vi "MainRIOJuan.vi"() -> ()   [LabVIEW 2020]
uses:
  Type Definitions/Acelerometer data--cluster.ctl
  Type Definitions/Shared.lvlib
  <vilib>/PantherLAB/Firebase API/PantherLAB_lib_Filtering Parameters--cluster.ctl
  <vilib>/PantherLAB/Firebase API/PantherLAB_lib_firebase.lvclass
  a087fea8-a487-4c1c-8a8b-15f205e78756.vi
  <vilib>/JDP Science/JSONtext/JSONtext.lvlib
  c90b4970-0cb1-4ed8-a3e8-abf7f56642d0.vi
  079ee137-338a-4224-8d27-3950f07d8dd5.vi
  Type Definitions/RIOData--cluster.ctl
panel:
  in  "Get All":bool
  in  "Get5":bool
  out "JSON String":string
  in  "Get Newest":bool
  in  "Delete":bool
  in  "Password":string
  in  "Email":string
  in  "Log In":bool
  in  "Sign In":bool
  out "Newest":T1
  out "Data out":T1[](array[typedef])
  out "My RIO Acelerometer":T2(graph)
  # "To add an authenticated user\nto your Real Time Database"
  # "If you are already authenticated\nand you want to start using\nyour Database"
  # "Warning:\nThis button will delete all the data\nunder Post EndPoint"
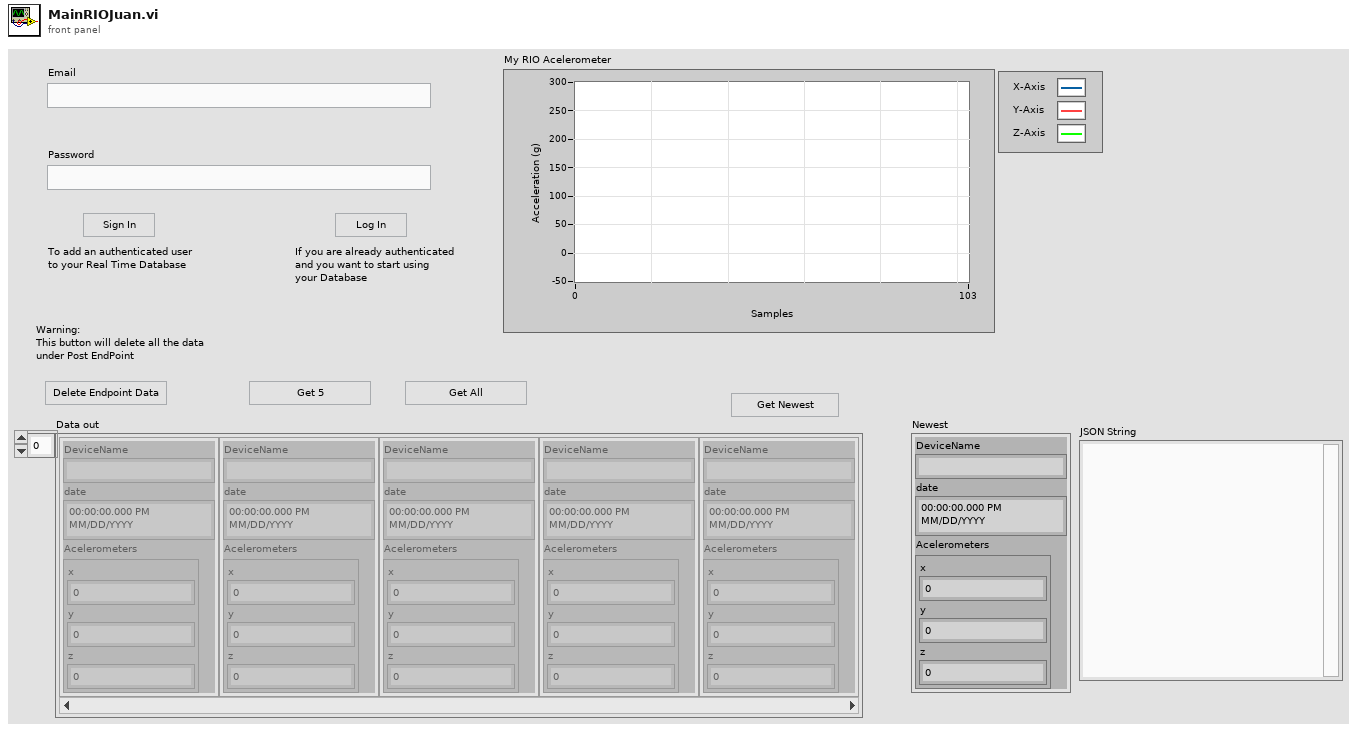
[diagram p1: front panel]
types:
  T1 = typedef "Shared.lvlib/RIOData--cluster.ctl" = cluster{"DeviceName":string, "date":timestamp, "Acelerometers":cluster{"x":dbl, "y":dbl, "z":dbl}}
  T2 = typedef "Shared.lvlib/Acelerometer data--cluster.ctl" = cluster{"X-Axis":dbl, "Y-Axis":dbl, "Z-Axis":dbl}
  T3 = cluster{"Read Access":enum8{"Allowed", "Required", "None"}, "Write Access":enum8{"Allowed", "Required", "None"}}
  T4 = typedef "PantherLAB_lib_firebase.lvclass/PantherLAB_lib_Filtering Parameters--cluster.ctl" = cluster{"Filtering Param":string, "Argument":string}
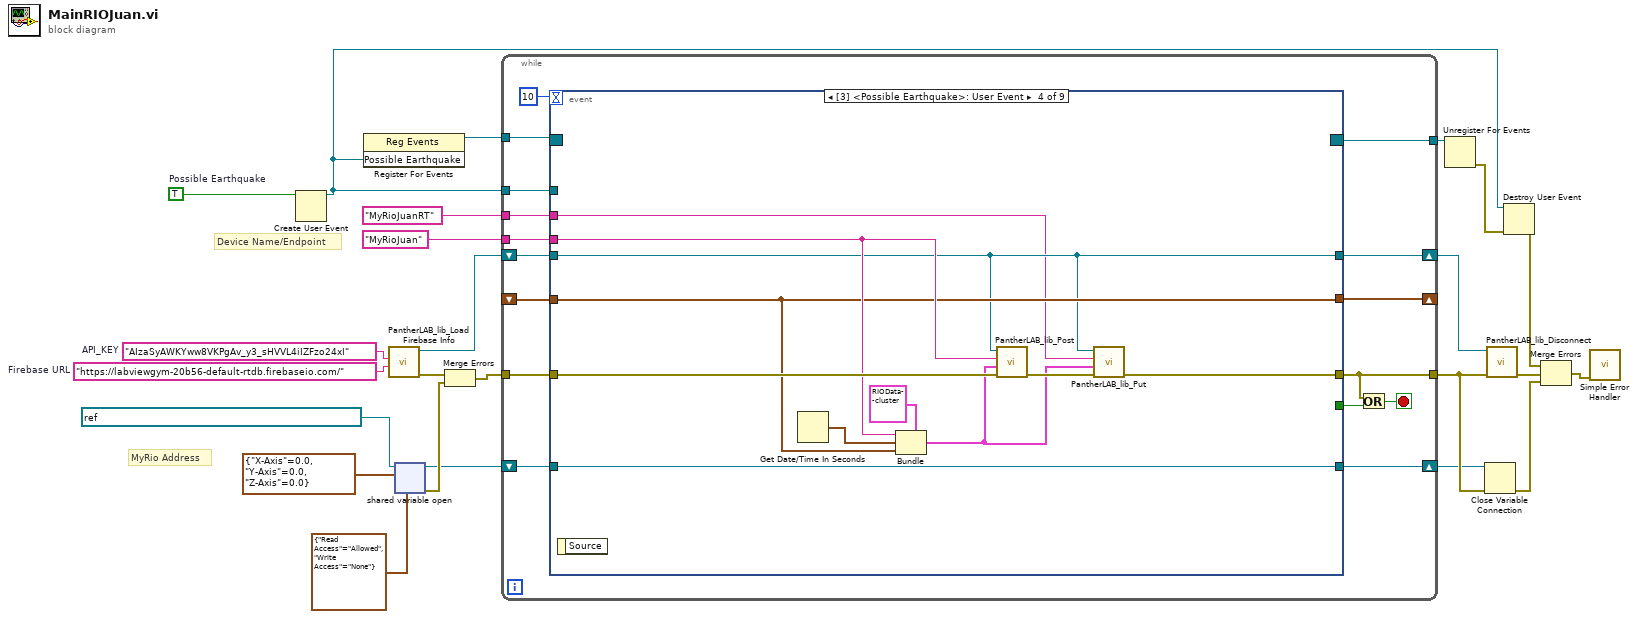
[diagram p0: block diagram]
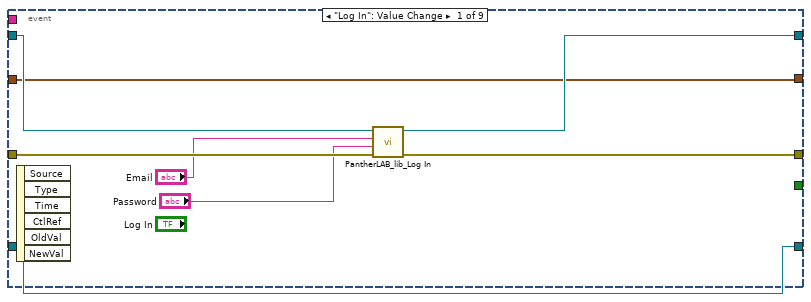
[diagram p2: hidden frame]
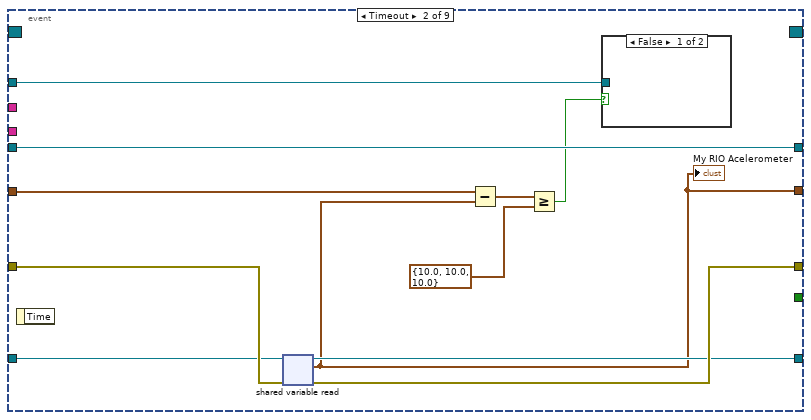
[diagram p3: hidden frame]
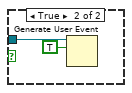
[diagram p4: hidden frame]
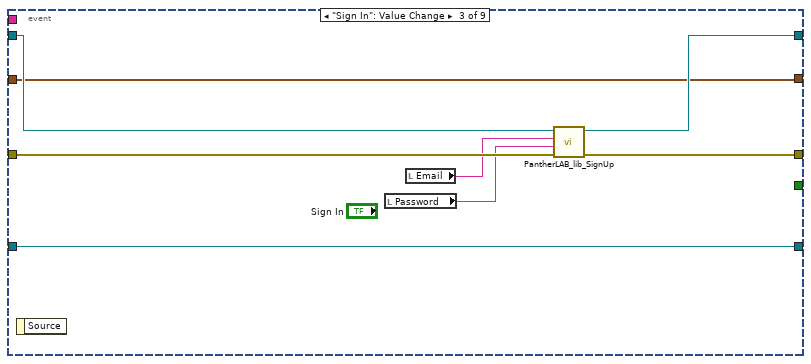
[diagram p5: hidden frame]
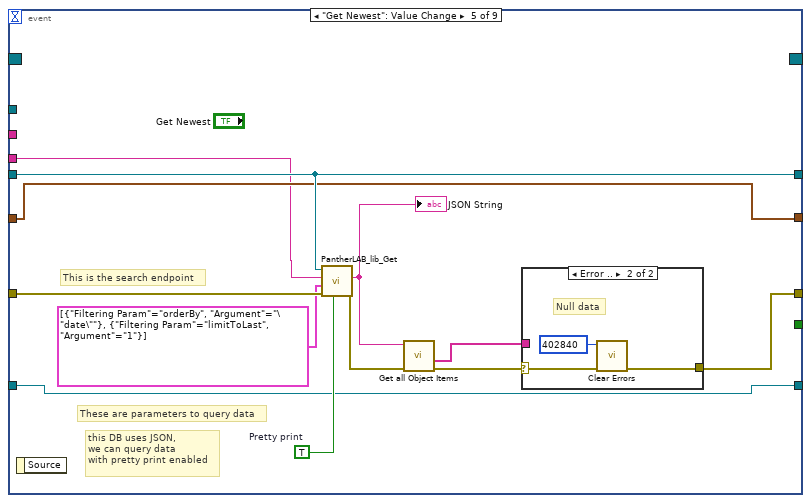
[diagram p6: hidden frame]
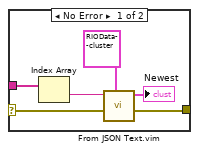
[diagram p7: hidden frame]
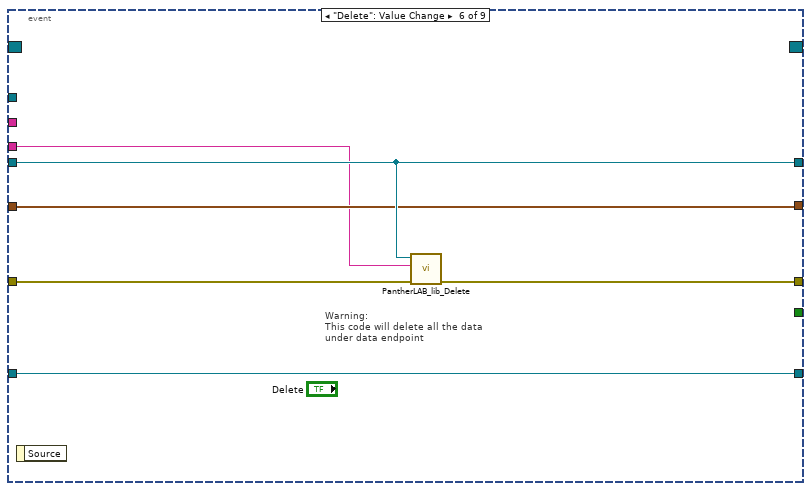
[diagram p8: hidden frame]
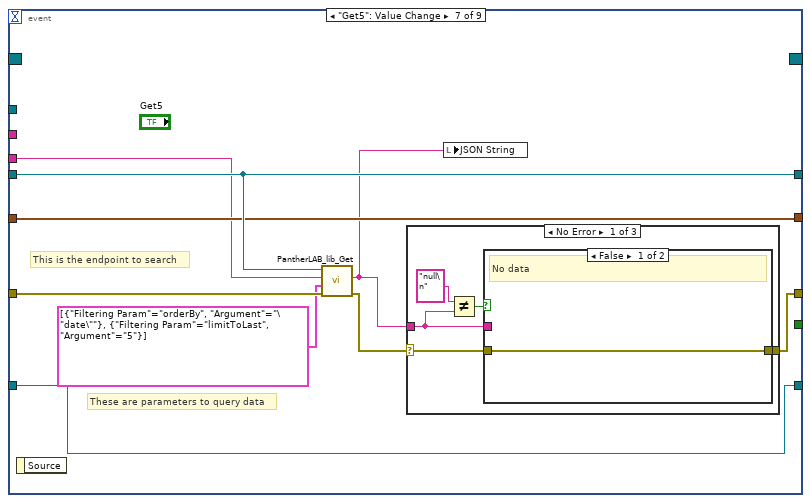
[diagram p9: hidden frame]
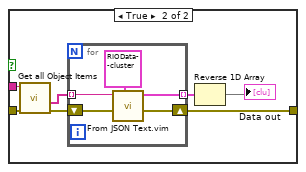
[diagram p10: hidden frame]
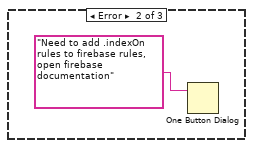
[diagram p11: hidden frame]
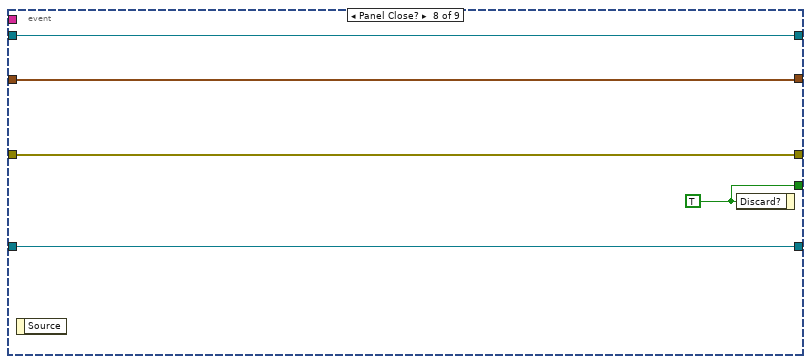
[diagram p13: hidden frame]
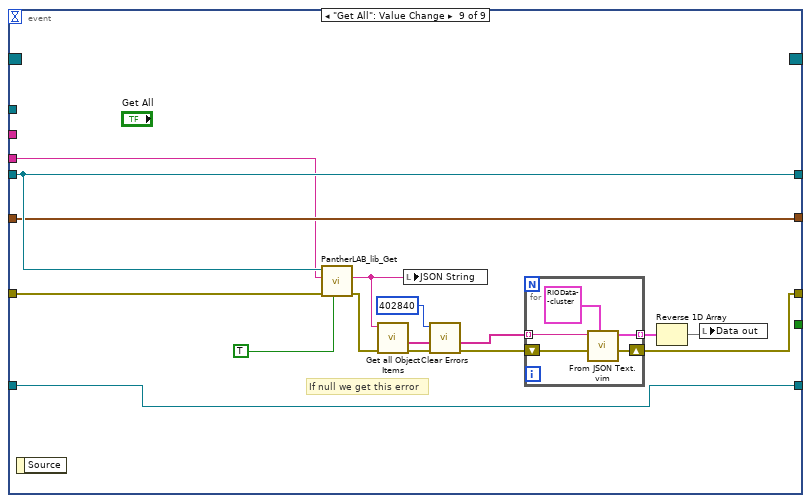
[diagram p14: hidden frame]
diagram:
  w5 = TRUE  # Possible Earthquake
  w10 = "AIzaSyAWKYww8VKPgAv_y3_sHVVL4iIZFzo24xI"  # API_KEY
  w9 = "https://labviewgym-20b56-default-rtdb.firebaseio.com/"  # Firebase URL
  # "MyRio Address"
  # "Device Name/Endpoint"
  n1 = Create User Event(user event datatype=w5) -> (user event=w3:refnum<user-event>)  [unwired: 1 in, 1 out]
  n2 = register-events(w3) -> (reference out=w6:refnum<event-registration>)  [unwired: 2 in, 1 out]
  n3 = call <vilib>:"PantherLAB_lib_Load Firebase Info.vi"("Firebase URL"=w9, "API_KEY"=w10) -> ("error out"=w23:errorcluster, "firebase out"=w11:refnum<class "PantherLAB_lib_firebase.lvclass">)  [unwired: 8 in]
  n4 = shared-variable-open(refnum<k21> "ni.var.psp://mjolnir/MyRIO Data/Accelerometer" ("shared variable refnum in"), T2 {"X-Axis"=0.0, "Y-Axis"=0.0, "Z-Axis"=0.0} ("Acceleration"), T3 {"Read Access"=enum."Allowed", "Write Access"=enum."None"} ("access")) -> (w8:refnum<k21>, w21:errorcluster)  [unwired: 1 in]
  n5 = Merge Errors(w23, w21) -> (w22:errorcluster)
  n6 = while {
    tunnel: w22 -> [w40]
    tunnel: [w39] -> w20
    shift-right: [w35] -> w12
    shift-left: w11 -> [w36]
    shift-right: [w32] -> w7
    shift-left: w8 -> [w33]
    tunnel: w6 -> [w31]
    tunnel: w3 -> [w30]
    shift-right: [w29] -> _
    shift-left: _ -> [w28]
    tunnel: [w27] -> w4
    tunnel: "MyRioJuan" -> [w26]
    tunnel: "MyRioJuanRT" -> [w25]
    stop <- w37 stop-if-true
    n7 = event shown="[3] <Possible Earthquake>: User Event" {
      selector: w31 -> [_ _ _ _ _ _ _ _ _]
      dyn-events: [_ _ _ _ _ _ _ _ _] -> w27
      timeout: 10 -> [_ _ _ _ _ _ _ _ _]
      tunnel: w40 -> [w48 w59 w69 w80 w92 w107 w116 w141 w156]
      tunnel: [w47 w58 w68 w73 w90 w106 w114 w141 w153] -> w39
      tunnel: [_ _ _ _ _ _ _ w139 _] -> w38
      tunnel: w36 -> [w44 w57 w65 w72 w86 w105 w112 w140 w146]
      tunnel: [w43 w57 w64 w72 w86 w105 w112 w140 w146] -> w35
      tunnel: w33 -> [w42 w56 w63 w78 w85 w104 w111 w138 w145]
      tunnel: [w42 w55 w63 w78 w85 w104 w111 w138 w145] -> w32
      tunnel: w30 -> [_ w52 _ _ _ _ _ _ _]
      tunnel: [w41 w50 w62 w74 w84 w103 w110 w137 w144] -> w29
      tunnel: w28 -> [w41 w51 w62 w74 w84 w103 w110 w137 w144]
      tunnel: w26 -> [_ _ _ w77 w83 w102 w109 _ w143]
      tunnel: w25 -> [_ _ _ w71 _ _ _ _ _]
      event "Log In": Value Change {
        n8 = event-data() -> ()  [unwired: 1 in, 6 out]
        n9 = call-dynamic "PantherLAB_lib_Log In.vi"("error in"=w48, "password"="Password", "email"="Email", "firebase in"=w44) -> ("error out"=w47:errorcluster, "firebase out"=w43:refnum<class "PantherLAB_lib_firebase.lvclass">)  [unwired: 6 in]
      }
      event Timeout {
        n10 = event-data() -> ()  [unwired: 1 in, 1 out]
        n11 = shared-variable-read(w56, w59) -> (w55:refnum<k21>, w58:errorcluster, w50:T2)  [unwired: 1 out]
        "My RIO Acelerometer" <- w50
        n12 = Subtract(x=w51, y=w50) -> (x-y=w54:T2)
        n13 = Greater Or Equal?(x=w54, y=T2 {"X-Axis"=10.0, "Y-Axis"=10.0, "Z-Axis"=10.0} ("x")) -> (x >= y?=w49:bool)
        n14 = case shown="False" w49 {
          tunnel: w52 -> [_ w61]
          frame False {
          }
          frame True {
            n15 = Generate User Event(user event=w61, event data cluster=TRUE ("event data")) -> ()  [unwired: 2 in, 2 out]
          }
        }
      }
      event "Sign In": Value Change {
        n16 = event-data() -> ()  [unwired: 1 in, 1 out]
        n17 = local read "Password"() -> (w67:string)
        n18 = local read "Email"() -> (w66:string)
        n19 = call-dynamic "PantherLAB_lib_SignUp.vi"("error in"=w69, "password"=w67, "email"=w66, "firebase in"=w65) -> ("error out"=w68:errorcluster, "firebase out"=w64:refnum<class "PantherLAB_lib_firebase.lvclass">)  [unwired: 6 in]
      }
      event User Event {
        n20 = event-data() -> ()  [unwired: 1 in, 1 out]
        n21 = Get Date/Time In Seconds() -> (seconds since 1Jan1904=w76:timestamp)
        n22 = Bundle(cluster=T1 {"DeviceName"="", "date"=timestamp(0 s since 1904-01-01), "Acelerometers"={"x"=0.0, "y"=0.0, "z"=0.0}} ("output cluster"), "DeviceName"=w77, "date"=w76, "Acelerometers"=w74) -> (w70:T1)
        n23 = call-dynamic "PantherLAB_lib_Post.vi"("error in"=w80, "Anything"=w70, "endPoint"=w77, "firebase in"=w72) -> ("error out"=w79:errorcluster)  [unwired: 6 in, 1 out]
        n24 = call-dynamic "PantherLAB_lib_Put.vi"("error in"=w79, "Anything"=w70, "endPoint"=w71, "firebase in"=w72) -> ("error out"=w73:errorcluster)  [unwired: 6 in, 1 out]
      }
      event "Get Newest": Value Change {
        w87 = TRUE  # Pretty print
        # "this DB uses JSON,\nwe can query data\nwith pretty print enabled"
        # "These are parameters to query data"
        # "This is the search endpoint"
        n25 = event-data() -> ()  [unwired: 1 in, 1 out]
        n26 = call-dynamic "PantherLAB_lib_Get.vi"("Pretty print"=w87, "error in"=w92, "Filtering Params"=T4[] [{"Filtering Param"="orderBy", "Argument"="\"date\""}, {"Filtering Param"="limitToLast", "Argument"="1"}], "endPoint"=w83, "firebase in"=w86) -> ("error out"=w91:errorcluster, "Json String"=w88:string)  [unwired: 5 in]
        "JSON String" <- w88
        n27 = call <vilib>:"Get all Object Items.vi"("error in (no error)"=w91, "JSON"=w88) -> ("error out"=w82:errorcluster, "<JSON>"=w81:string[])  [unwired: 6 in, 2 out]
        n28 = case shown="Error .." w82 {
          selector: w82 -> [w98 w101]
          tunnel: [w97 w100] -> w90
          tunnel: w81 -> [w96 _]
          frame No Error {
            n29 = Index Array(array=w96) -> (element=w95:string)  [unwired: 1 in]
            n30 = call "From JSON Text.vim"("Data Type and Default Value"=T1 {"DeviceName"="", "date"=timestamp(0 s since 1904-01-01), "Acelerometers"={"x"=0.0, "y"=0.0, "z"=0.0}} ("Array"), "error in (no error)"=w98, "JSON"=w95) -> ("error out"=w97:errorcluster, "Data out"=→"Newest":T1)  [unwired: 7 in]
          }
          frame Error {
            # "Null data"
            n31 = call <vilib>:"Clear Errors.vi"("error in (no error)"=w101, "specific error code to clear (0: all)"=402840) -> ("error out"=w100:errorcluster)  [unwired: 4 in, 1 out]
          }
        }
      }
      event "Delete": Value Change {
        # "Warning:\nThis code will delete all the data\nunder data endpoint"
        n32 = event-data() -> ()  [unwired: 1 in, 1 out]
        n33 = call-dynamic "PantherLAB_lib_Delete.vi"("error in"=w107, "endPoint"=w102, "firebase in"=w105) -> ("error out"=w106:errorcluster)  [unwired: 7 in, 1 out]
      }
      event "Get5": Value Change {
        # "This is the endpoint to search"
        # "These are parameters to query data"
        n34 = event-data() -> ()  [unwired: 1 in, 1 out]
        n35 = call-dynamic "PantherLAB_lib_Get.vi"("error in"=w116, "Filtering Params"=T4[] [{"Filtering Param"="orderBy", "Argument"="\"date\""}, {"Filtering Param"="limitToLast", "Argument"="5"}], "endPoint"=w109, "firebase in"=w112) -> ("error out"=w115:errorcluster, "Json String"=w108:string)  [unwired: 6 in]
        n36 = case shown="No Error" w115 {
          selector: w115 -> [w121 _ w136]
          tunnel: [w120 _ w136] -> w114
          tunnel: w108 -> [w117 _ _]
          frame No Error {
            n37 = Not Equal?(x="null\n" ("Display"), y=w117) -> (x != y?=w118:bool)
            n38 = case shown="False" w118 {
              tunnel: w121 -> [w122 w128]
              tunnel: [w122 w127] -> w120
              tunnel: w117 -> [_ w124]
              frame False {
                # "No data"
              }
              frame True {
                n39 = call <vilib>:"Get all Object Items.vi"("error in (no error)"=w128, "JSON"=w124) -> ("error out"=w129:errorcluster, "<JSON>"=w126:string[])  [unwired: 6 in, 2 out]
                n40 = for {
                  tunnel: w126 -> [w132] mode=indexing
                  shift-right: [w133] -> w127
                  shift-left: w129 -> [w134]
                  tunnel: [w131] -> w125 mode=indexing
                  n41 = call "From JSON Text.vim"("Data Type and Default Value"=T1 {"DeviceName"="", "date"=timestamp(0 s since 1904-01-01), "Acelerometers"={"x"=0.0, "y"=0.0, "z"=0.0}} ("RioData"), "error in (no error)"=w134, "JSON"=w132) -> ("error out"=w133:errorcluster, "Data out"=w131:T1)  [unwired: 7 in]
                }
                n42 = Reverse 1D Array(array=w125) -> (reversed array=→"Data out":T1[])
              }
            }
          }
          frame Error {
            n43 = One Button Dialog(message="Need to add .indexOn rules to firebase rules, open firebase documentation") -> ()  [unwired: 1 in, 1 out]
          }
          frame Default {
          }
        }
        n44 = local write "JSON String"(w108) -> ()
      }
      event Panel Close? {
        w139 = TRUE ("Discard?")
        n45 = event-data() -> ()  [unwired: 1 in, 1 out]
        n46 = event-data("Discard?"=w139) -> ()  [unwired: 1 in, 1 out]
      }
      event "Get All": Value Change {
        # "If null we get this error"
        n47 = event-data() -> ()  [unwired: 1 in, 1 out]
        n48 = call-dynamic "PantherLAB_lib_Get.vi"("Pretty print"=TRUE, "error in"=w156, "endPoint"=w143, "firebase in"=w146) -> ("error out"=w154:errorcluster, "Json String"=w149:string)  [unwired: 6 in]
        n49 = call <vilib>:"Get all Object Items.vi"("error in (no error)"=w154, "JSON"=w149) -> ("error out"=w155:errorcluster, "<JSON>"=w151:string[])  [unwired: 6 in, 2 out]
        n50 = local write "JSON String"(w149) -> ()
        n51 = call <vilib>:"Clear Errors.vi"("error in (no error)"=w155, "specific error code to clear (0: all)"=402840) -> ("error out"=w152:errorcluster)  [unwired: 4 in, 1 out]
        n52 = for {
          tunnel: w151 -> [w159] mode=indexing
          shift-right: [w160] -> w153
          shift-left: w152 -> [w161]
          tunnel: [w158] -> w150 mode=indexing
          n53 = call "From JSON Text.vim"("Data Type and Default Value"=T1 {"DeviceName"="", "date"=timestamp(0 s since 1904-01-01), "Acelerometers"={"x"=0.0, "y"=0.0, "z"=0.0}} ("RioData"), "error in (no error)"=w161, "JSON"=w159) -> ("error out"=w160:errorcluster, "Data out"=w158:T1)  [unwired: 7 in]
        }
        n54 = Reverse 1D Array(array=w150) -> (reversed array=w142:T1[])
        n55 = local write "Data out"(w142) -> ()
      }
    }
    n56 = Or(x=w39, y=w38) -> (x .or. y?=w37:bool)
  }
  n57 = Unregister For Events(event registration refnum=w4) -> (error out=w16:errorcluster)  [unwired: 1 in]
  n58 = Close Variable Connection(8:w20, 11:w7) -> (0:w18:errorcluster)
  n59 = call-dynamic "PantherLAB_lib_Disconnect.vi"("error in"=w20, "firebase in"=w12) -> ("error out"=w24:errorcluster)  [unwired: 9 in]
  n60 = Destroy User Event(user event=w3, error in=w16) -> (error out=w17:errorcluster)
  n61 = Merge Errors(w17, w24, w18) -> (w19:errorcluster)
  n62 = call <vilib>:"Simple Error Handler.vi"("error in (no error)"=w19) -> ()  [unwired: 4 in, 5 out]
